vi "InstrQuery.vi"(8 "error in (no error)":errorcluster, 10 "Command string":string, 11 "InstControl in":refnum<class "InstrControl.lvclass">) -> (0 "error out":errorcluster, 2 "Instrument response":string, 3 "InstControl out":refnum<class "InstrControl.lvclass">)   [LabVIEW 2013, in "InstrControl.lvclass"]
uses:
  InstrControl.lvclass
  InstrControl.lvclass/InstrControl.ctl
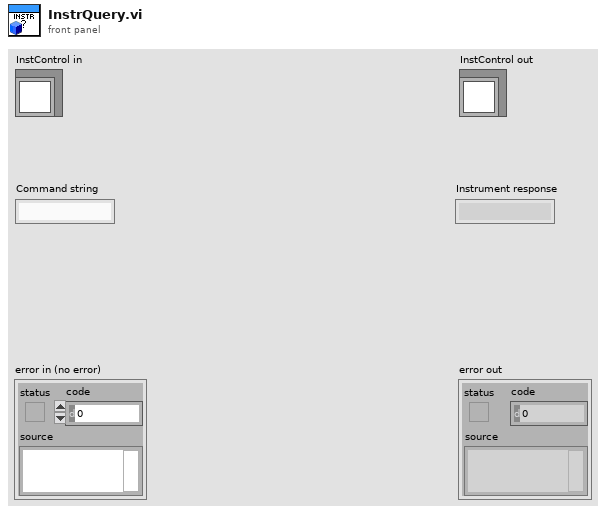
[diagram p1: front panel]
types:
  T1 = cluster{"error":bool, "code":i32, "source":string}
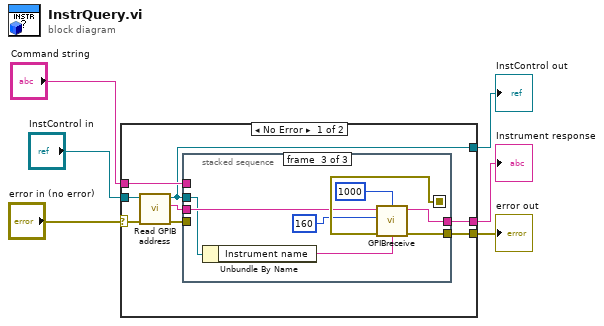
[diagram p0: block diagram]
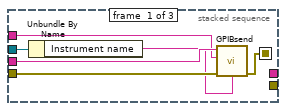
[diagram p2: hidden frame]
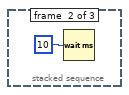
[diagram p3: hidden frame]
diagram:
  n1 = case shown="No Error" "error in (no error)" {
    selector: "error in (no error)" -> [w10 w31]
    tunnel: [w14 w31] -> w5
    tunnel: [w7 w30] -> w3
    tunnel: "InstControl in" -> [w12 w30]
    tunnel: "Command string" -> [w13 _]
    tunnel: [w8 _] -> w1
    frame No Error {
      n2 = call-dynamic "Read GPIB address.vi"("error in (no error)"=w10, "InstControl in"=w12) -> ("error out"=w9:errorcluster, "GPIB address"=w11:string, "InstControl out"=w7:refnum<class "InstrControl.lvclass">)  [unwired: 7 in]
      n3 = stacked-sequence {
        seq-local: [w17 _ _] -> [_ _ w28]
        tunnel: w11 -> [w20 _ w27]
        tunnel: w9 -> [w19 _ _]
        tunnel: [_ _ w29] -> w14
        tunnel: w13 -> [w18 _ _]
        tunnel: [_ _ w25] -> w8
        tunnel: w7 -> [w16 _ w24]
        frame #0 {
          n4 = Unbundle By Name(w16) -> ("Instrument name"=w15:string)
          n5 = call "GPIBsend.vi"("address string"=w20, "write buffer"=w18, "source"=w15, "error in"=w19) -> ("error out"=w17:errorcluster)  [unwired: 3 in, 2 out]
        }
        frame #1 {
          n6 = Wait (ms)(milliseconds to wait=10) -> ()  [unwired: 1 out]
        }
        frame #2 {
          n7 = Unbundle By Name(w24) -> ("Instrument name"=w23:string)
          n8 = call "GPIBreceive.vi"("timeout ms"=1000, "address string"=w27, "byte count"=160, "source"=w23, "error in"=w28) -> ("read buffer"=w25:string, "error out"=w29:T1)  [unwired: 2 in, 1 out]
        }
      }
    }
    frame Error {
    }
  }
  "error out" <- w5
  "InstControl out" <- w3
  "Instrument response" <- w1
